vi "Create_event_log_file.vi"(8 "error in":errorcluster) -> (0 "error out":errorcluster, 3 "Log file refnum out":refnum<file>, 5 "New log file path":path)   [LabVIEW 2017, in "labview-standard-library.lvlib" / "data-logging.lvlib"]
uses:
  data-logging.lvlib
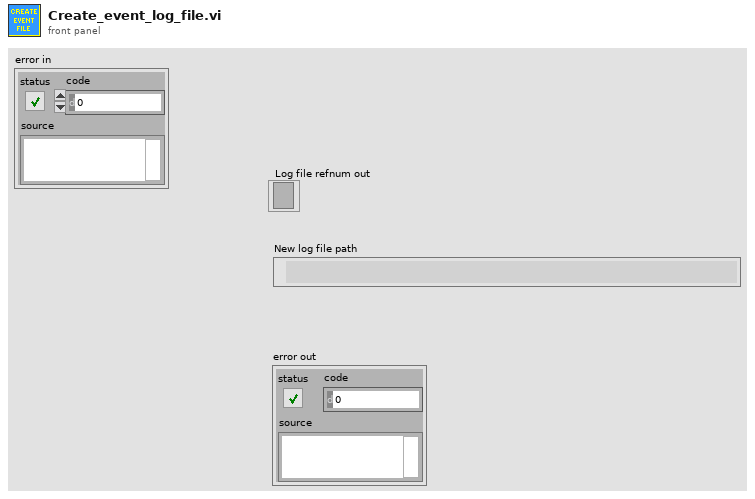
[diagram p1: front panel]
types:
  T1 = enum16{"open", "replace", "create", "open or create", "replace or create", "replace or create with confirmation"}
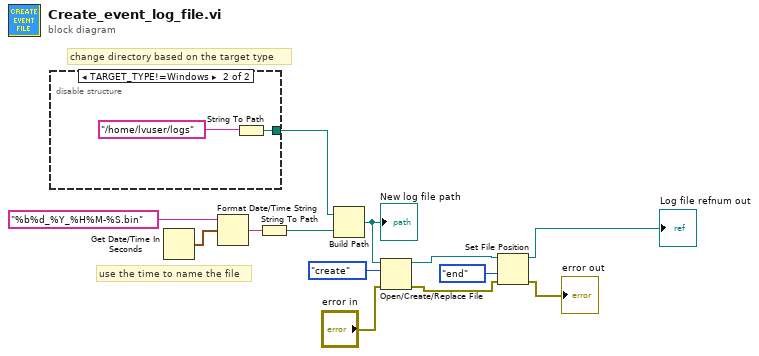
[diagram p0: block diagram]
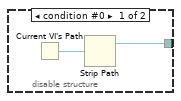
[diagram p2: hidden frame]
diagram:
  # "change directory based on the target type"
  # "use the time to name the file"
  n1 = disable-structure shown="TARGET_TYPE!=Windows" {
    disable-tunnel: [w14 w16] -> w12
    frame condition #0 {
      n2 = Current VI's Path() -> (path=w15:path)
      n3 = Strip Path(path=w15) -> (stripped path=w14:path)  [unwired: 1 out]
    }
    frame condition #1 (active) {
      n4 = String To Path(string="/home/lvuser/logs") -> (path=w16:path)
    }
  }
  n5 = Get Date/Time In Seconds() -> (seconds since 1Jan1904=w13:timestamp)
  n6 = Format Date/Time String(time format string (%c)="%b%d_%Y_%H%M-%S.bin", seconds (now)=w13) -> (date/time string=w10:string)  [unwired: 1 in]
  n7 = String To Path(string=w10) -> (path=w11:path)
  n8 = Build Path(base path=w12, name or relative path=w11) -> (appended path=w8:path)
  "New log file path" <- w8
  n9 = Open/Create/Replace File(file path (use dialog)=w8, error in="error in", operation (0:open)=T1."create") -> (refnum out=w4:refnum<file>, error out=w5:errorcluster)  [unwired: 3 in, 1 out]
  n10 = Set File Position(refnum=w4, from (0:start)=enum16{"start", "end", "current"}."end", error in=w5) -> (refnum out=→"Log file refnum out":refnum<file>, error out=→"error out":errorcluster)  [unwired: 1 in]
